vi "DriveSimulationExecute.vi"(6 "GyroStatus":T7, 8 "error in (no error)":errorcluster, 9 "GyroValuesDeg":T8, 10 "ModulePositions":T1[](array[typedef]) {"Angle"."SIN" format="%13.4f"; "Angle"."COS" format="%13.4f"; "Angle"."VALUE" format="%13.4f"}, 11 "ModuleStates":T6[](array[typedef]) {"Angle"."SIN" format="%13.4f"; "Angle"."COS" format="%13.4f"; "Angle"."VALUE" format="%13.4f"}) -> (0 "error out":errorcluster, 1 "outModulePositions":T1[](array[typedef]) {"Angle"."SIN" format="%13.4f"; "Angle"."COS" format="%13.4f"; "Angle"."VALUE" format="%13.4f"}, 2 "SpinMotorDmds":dbl[](array[numeric]), 3 "TravelMotorDmds":dbl[](array[numeric]), 5 "out SWERVE_DRIVE_KINEMATICS":T3 {"SavedModuleStates"."Angle"."SIN" format="%13.4f"; "SavedModuleStates"."Angle"."COS" format="%13.4f"; "SavedModuleStates"."Angle"."VALUE" format="%13.4f"; "PrevCoR"."Y" format="%14.3f"; "PrevCoR"."X" format="%14.3f"; "Modules"."Y" format="%14.3f"; "Modules"."X" format="%14.3f"})   [LabVIEW 2023]
doc: "Execute for Drie\n\nClosed control loop for drive\n\ninput: \n error in (cluster)\n\noutput:\n error out (cluster)"
uses:
  <vilib>/Rock Robotics/WPI/ThirdParty/JAS_Junk/TrajLib/TypeDef/SWERVE_DRIVE_MODULE_STATE.ctl
  <vilib>/Rock Robotics/WPI/ThirdParty/ADI/ADIS16470/Typedef/ADIS16470 Data.ctl
  <vilib>/Rock Robotics/WPI/ThirdParty/ADI/ADIS16470/Typedef/ADIS16470 Status.ctl
  <vilib>/Rock Robotics/WPI/ThirdParty/JAS_Junk/TrajLib/TypeDef/SWERVE_DRIVE_KINEMATICS.ctl
  <vilib>/Analysis/Matrix/Datatypes/RealMatrix.ctl
  <vilib>/Rock Robotics/WPI/ThirdParty/JAS_Junk/TrajLib/TypeDef/TRANSLATION2D.ctl
  <vilib>/Rock Robotics/WPI/ThirdParty/JAS_Junk/TrajLib/LinearFilter_LP_BW1_Execute.vi
  <vilib>/Rock Robotics/WPI/ThirdParty/JAS_Junk/TrajLib/LinearFilter_ResetToValue.vi
  <vilib>/Rock Robotics/WPI/ThirdParty/JAS_Junk/TrajLib/LinearFilter_Calculate.vi
  <vilib>/Rock Robotics/WPI/ThirdParty/JAS_Junk/TrajLib/Conv_Deg_Radians.vi
  <vilib>/Rock Robotics/WPI/ThirdParty/JAS_Junk/TrajLib/Rotation2d_CreateAngle.vi
  <vilib>/Rock Robotics/WPI/ThirdParty/JAS_Junk/TrajLib/VI/Util_GetTime_U32.vi
  <vilib>/Rock Robotics/WPI/ThirdParty/JAS_Junk/TrajLib/Conv_Feet_Meters.vi
  DriveGetMaxSpeed.vi
  <vilib>/Rock Robotics/WPI/ThirdParty/JAS_Junk/TrajLib/SwerveModuleState_Optimize.vi
  <vilib>/Rock Robotics/WPI/ThirdParty/JAS_Junk/TrajLib/ControllerUtil_GetModulusError.vi
  GeneralPurpose/PositionControl.vi
  <vilib>/Rock Robotics/WPI/ThirdParty/JAS_Junk/TrajLib/SimpleMotorFF_New.vi
  <vilib>/Rock Robotics/WPI/ThirdParty/JAS_Junk/TrajLib/SimpleMotorFF_Calculate_CalcAccel.vi
  <vilib>/Rock Robotics/WPI/ThirdParty/JAS_Junk/TrajLib/PIDController_AdvExecute.vi
  <vilib>/Rock Robotics/WPI/ThirdParty/JAS_Junk/TrajLib/PIDController_Pack_AdvLimits.vi
  <vilib>/Rock Robotics/WPI/ThirdParty/JAS_Junk/TrajLib/PIDController_Pack_AdvTuning.vi
  <vilib>/Rock Robotics/WPI/ThirdParty/JAS_Junk/TrajLib/SlewRateLimiter_Execute.vi
  GeneralPurpose/Robot_Enabled.vi
  <vilib>/Rock Robotics/WPI/ThirdParty/JAS_Junk/TrajLib/Rotation2d_Minus.vi
  <vilib>/Rock Robotics/WPI/ThirdParty/JAS_Junk/TrajLib/Rotation2d_GetRadians.vi
  <vilib>/Rock Robotics/WPI/ThirdParty/JAS_Junk/TrajLib/SwerveModuleState_New.vi
  <vilib>/Rock Robotics/WPI/ThirdParty/JAS_Junk/TrajLib/Rotation2d_RotateBy.vi
  <vilib>/Rock Robotics/WPI/ThirdParty/JAS_Junk/TrajLib/SimpleMotorFF_Calculate.vi
  <vilib>/Rock Robotics/WPI/ThirdParty/JAS_Junk/TrajLib/PIDController_AtSetpoint.vi
  <vilib>/Rock Robotics/WPI/ThirdParty/JAS_Junk/TrajLib/PIDController_SetPIDF.vi
  <vilib>/Rock Robotics/WPI/ThirdParty/JAS_Junk/TrajLib/PIDController_SetDerivativeFilter.vi
  <vilib>/Rock Robotics/WPI/ThirdParty/JAS_Junk/TrajLib/PIDController_SetIntegratorRange.vi
  <vilib>/Rock Robotics/WPI/ThirdParty/JAS_Junk/TrajLib/PIDController_SetTolerancePandV.vi
  <vilib>/Rock Robotics/WPI/ThirdParty/JAS_Junk/TrajLib/PIDController_DisableContinousInput.vi
  <vilib>/Rock Robotics/WPI/ThirdParty/JAS_Junk/TrajLib/PIDController_EnableContinousInput.vi
  <vilib>/Rock Robotics/WPI/ThirdParty/JAS_Junk/TrajLib/PIDController_Reset.vi
  <vilib>/Rock Robotics/WPI/ThirdParty/JAS_Junk/TrajLib/PIDController_New.vi
  <vilib>/Rock Robotics/WPI/ThirdParty/JAS_Junk/TrajLib/PIDController_SetOutputLimits.vi
  <vilib>/Rock Robotics/WPI/ThirdParty/JAS_Junk/TrajLib/VI/PIDController_SetIntegratorZone.vi
  <vilib>/Rock Robotics/WPI/ThirdParty/JAS_Junk/TrajLib/SlewRateLimiter_New.vi
  <vilib>/Rock Robotics/WPI/ThirdParty/JAS_Junk/TrajLib/SlewRateLimiter_Reset.vi
  <vilib>/Rock Robotics/WPI/ThirdParty/JAS_Junk/TrajLib/SlewRateLimiter_Calculate.vi
  <vilib>/Rock Robotics/WPI/ThirdParty/JAS_Junk/TrajLib/SlewRateLimiter_SetRate.vi
  <vilib>/Rock Robotics/WPI/ThirdParty/JAS_Junk/TrajLib/Rotation2d_UnaryMinus.vi
  <vilib>/Rock Robotics/WPI/ThirdParty/JAS_Junk/TrajLib/Rotation2d_CreateXY.vi
  <vilib>/Rock Robotics/WPI/ThirdParty/JAS_Junk/TrajLib/PIDController_NewPeriod.vi
  <vilib>/Rock Robotics/WPI/ThirdParty/JAS_Junk/TrajLib/Util_CalcDist.vi
  <vilib>/Rock Robotics/SystemInterfaces/NetworkCommunication/NetComm_UsageReport_report.vi
  DriveGlobal.vi
  <vilib>/Rock Robotics/WPI/ThirdParty/JAS_Junk/TrajLib/LinearFilter_LowPassBW1.vi
  <vilib>/Rock Robotics/WPI/ThirdParty/JAS_Junk/TrajLib/VI/Util_GetTime_U64.vi
  Robot Global Data.vi
  <vilib>/Rock Robotics/WPI/ThirdParty/JAS_Junk/TrajLib/Globals/Util_LibraryGlobals.vi
  <vilib>/Rock Robotics/WPI/ThirdParty/JAS_Junk/TrajLib/PIDController_AdvCalculate_FF_Sp_Pv.vi
  <vilib>/Rock Robotics/WPI/ThirdParty/JAS_Junk/TrajLib/Trajectory_Library.lvlib
  <vilib>/Rock Robotics/WPI/ThirdParty/JAS_Junk/TrajLib/TypeDef/ROTATION2D.ctl
  <vilib>/Rock Robotics/WPI/ThirdParty/JAS_Junk/TrajLib/TypeDef/SWERVE_DRIVE_MODULE_POSITION.ctl
  <vilib>/Analysis/Matrix/NI_Matrix.lvlib
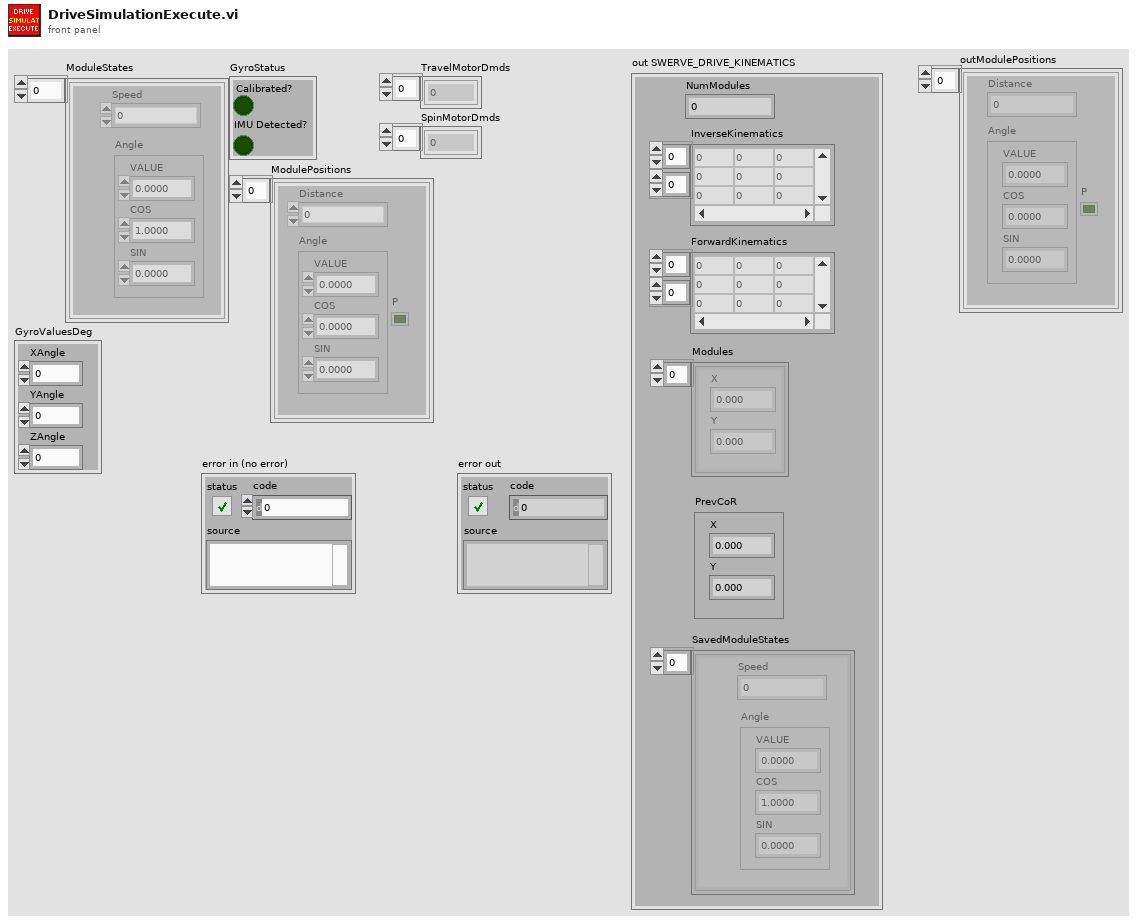
[diagram p1: front panel]
types:
  T1 = typedef "Trajectory_Library.lvlib/SWERVE_DRIVE_MODULE_POSITION.ctl" = cluster{"Distance":dbl, "Angle":T2, "P":bool}
  T2 = typedef "Trajectory_Library.lvlib/ROTATION2D.ctl" = cluster{"VALUE":dbl, "COS":dbl, "SIN":dbl}
  T3 = typedef "Trajectory_Library.lvlib/SWERVE_DRIVE_KINEMATICS.ctl" = cluster{"NumModules":i32, "InverseKinematics":T4, "ForwardKinematics":T4, "Modules":T5[], "PrevCoR":T5, "SavedModuleStates":T6[]}
  T4 = typedef "NI_Matrix.lvlib/RealMatrix.ctl" = dbl[][]
  T5 = typedef "Trajectory_Library.lvlib/TRANSLATION2D.ctl" = cluster{"X":dbl, "Y":dbl}
  T6 = typedef "Trajectory_Library.lvlib/SWERVE_DRIVE_MODULE_STATE.ctl" = cluster{"Speed":dbl, "Angle":T2}
  T7 = typedef "ADIS16470 Status.ctl" = cluster{"Calibrated?":bool, "IMU Detected?":bool}
  T8 = typedef "ADIS16470 Data.ctl" = cluster{"XAngle":dbl, "YAngle":dbl, "ZAngle":dbl}
  T9 = typedef "Trajectory_Library.lvlib/CHASSIS_SPEEDS.ctl" = cluster{"vX":dbl, "vY":dbl, "vOmega":dbl}
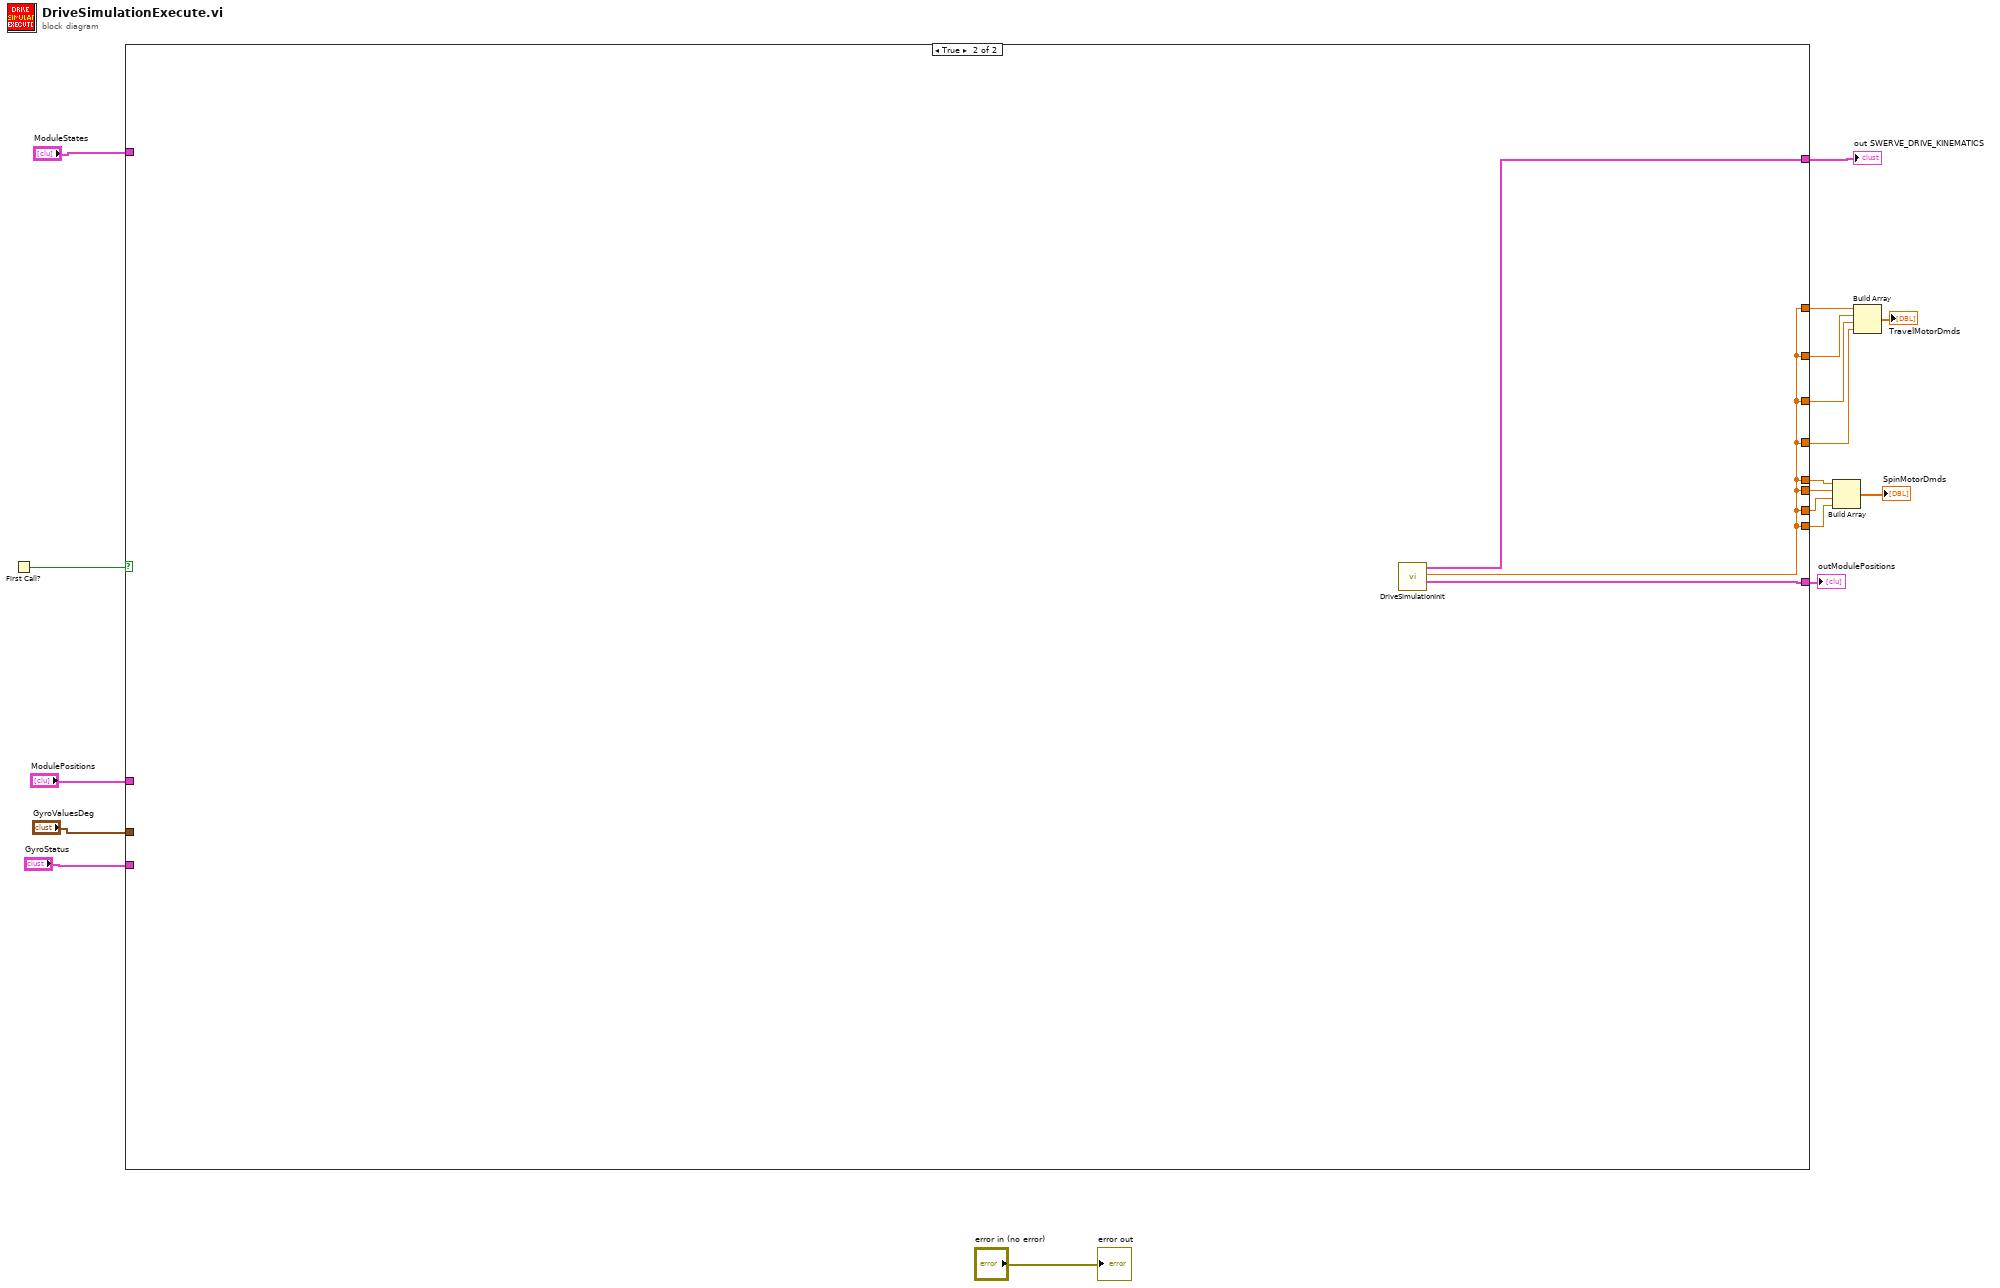
[diagram p0: block diagram]
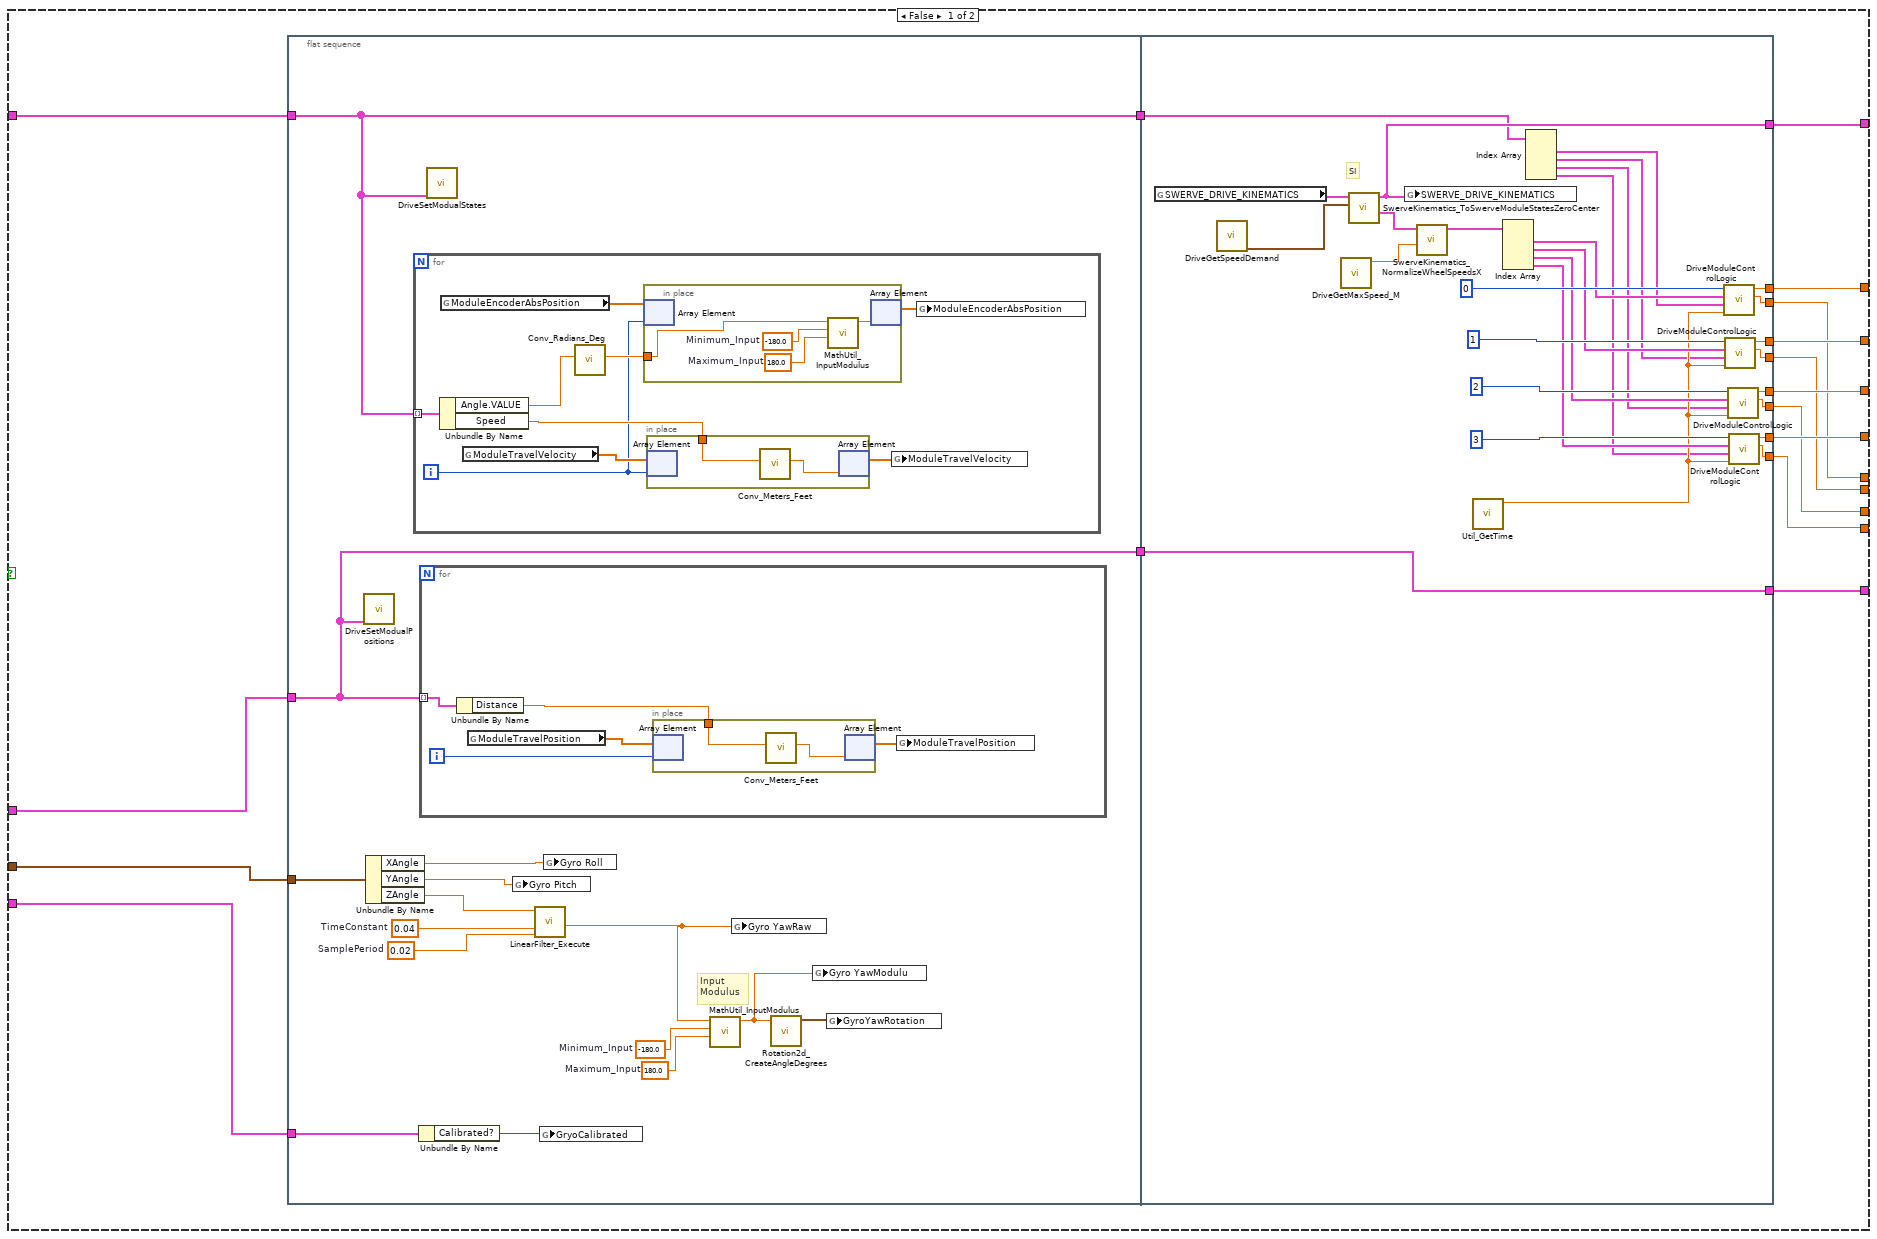
[diagram p2: hidden frame]
diagram:
  n1 = First Call?() -> (First Call?: T/F=w17:bool)
  n2 = case shown="True" w17 {
    tunnel: "ModuleStates" -> [w29 _]
    tunnel: "ModulePositions" -> [w23 _]
    tunnel: "GyroValuesDeg" -> [w22 _]
    tunnel: "GyroStatus" -> [w21 _]
    tunnel: [w28 w103] -> w10
    tunnel: [w26 w103] -> w9
    tunnel: [w25 w103] -> w8
    tunnel: [w24 w103] -> w7
    tunnel: [w34 w103] -> w6
    tunnel: [w33 w103] -> w5
    tunnel: [w32 w103] -> w4
    tunnel: [w31 w103] -> w3
    tunnel: [w30 w102] -> w2
    tunnel: [w20 w101] -> w1
    frame False {
      n3 = flat-sequence {
        tunnel: w29 -> [w49]
        tunnel: [w49] -> w27
        tunnel: w23 -> [w35]
        tunnel: w22 -> [w38]
        tunnel: w21 -> [w36]
        tunnel: [w35] -> w19
        tunnel: [w82] -> w26
        tunnel: [w81] -> w25
        tunnel: [w80] -> w24
        tunnel: [w79] -> w34
        tunnel: [w78] -> w33
        tunnel: [w77] -> w32
        tunnel: [w76] -> w31
        tunnel: [w75] -> w30
        tunnel: [w73] -> w28
        tunnel: w27 -> [w74]
        tunnel: [w72] -> w20
        tunnel: w19 -> [w72]
        frame #0 {
          w41 = -180.0  # Minimum_Input
          w42 = 180.0  # Maximum_Input
          w40 = 0.02  # SamplePeriod
          w39 = 0.04  # TimeConstant
          # "Input\nModulus"
          n4 = call "DriveSetModualPositions.vi"("Swerve_Drive_Modual_Position"=w35) -> ()  [unwired: 11 in]
          n5 = Unbundle By Name(w38) -> ("XAngle"=w48:dbl, "YAngle"=w47:dbl, "ZAngle"=w45:dbl)
          n6 = for {
            tunnel: w49 -> [w63] mode=indexing
            i -> [w58]
            n7 = Unbundle By Name(w63) -> ("Angle.VALUE"=w57:dbl, "Speed"=w62:dbl)
            n8 = global read "DriveGlobal.vi" "ModuleEncoderAbsPosition"() -> (w61:dbl[])
            n9 = global read "DriveGlobal.vi" "ModuleTravelVelocity"() -> (w65:dbl[])
            n10 = call <vilib>:"Conv_Radians_Deg.vi"("Radians"=w57) -> ("Degrees"=w59:dbl)  [unwired: 10 in]
            n11 = in-place {
              in-place-border: w59 -> [w66]
              w69 = -180.0  # Minimum_Input
              w68 = 180.0  # Maximum_Input
              n12 = in-place-array #1(w61, w58) -> ()  [unwired: 1 out]
              n13 = call <vilib>:"MathUtil_InputModulus.vi"("Maximum_Input"=w68, "Minimum_Input"=w69, "Input"=w66) -> ("modulus"=w67:dbl)  [unwired: 8 in]
              n14 = in-place-array #1(w67) -> (w60:dbl[])  [unwired: 1 out]
            }
            n15 = in-place {
              in-place-border: w62 -> [w70]
              n16 = in-place-array #2(w65, w58) -> ()  [unwired: 1 out]
              n17 = call <vilib>:"Conv_Meters_Feet.vi"("Meters"=w70) -> ("Feet"=w71:dbl)  [unwired: 10 in]
              n18 = in-place-array #2(w71) -> (w64:dbl[])  [unwired: 1 out]
            }
            n19 = global write "DriveGlobal.vi" "ModuleTravelVelocity"(w64) -> ()
            n20 = global write "DriveGlobal.vi" "ModuleEncoderAbsPosition"(w60) -> ()
          }
          n21 = Unbundle By Name(w36) -> ("Calibrated?"=w37:bool)
          n22 = for {
            tunnel: w35 -> [w52] mode=indexing
            i -> [w50]
            n23 = Unbundle By Name(w52) -> ("Distance"=w51:dbl)
            n24 = global read "DriveGlobal.vi" "ModuleTravelPosition"() -> (w54:dbl[])
            n25 = in-place {
              in-place-border: w51 -> [w55]
              n26 = in-place-array #3(w54, w50) -> ()  [unwired: 1 out]
              n27 = call <vilib>:"Conv_Meters_Feet.vi"("Meters"=w55) -> ("Feet"=w56:dbl)  [unwired: 10 in]
              n28 = in-place-array #3(w56) -> (w53:dbl[])  [unwired: 1 out]
            }
            n29 = global write "DriveGlobal.vi" "ModuleTravelPosition"(w53) -> ()
          }
          n30 = call "DriveSetModualStates.vi"("Swerve__Drive_Modual_States"=w49) -> ()  [unwired: 11 in]
          n31 = global write "DriveGlobal.vi" "Gyro Pitch"(w47) -> ()
          n32 = call-poly <vilib>:"LinearFilter_Execute.vi"("SamplePeriod"=w40, "TimeConstant"=w39, "Input"=w45) -> ("Output"=w46:dbl)  [unwired: 8 in]
          n33 = global write "DriveGlobal.vi" "GryoCalibrated"(w37) -> ()
          n34 = global write "DriveGlobal.vi" "Gyro Roll"(w48) -> ()
          n35 = call <vilib>:"MathUtil_InputModulus.vi"("Maximum_Input"=w42, "Minimum_Input"=w41, "Input"=w46) -> ("modulus"=w44:dbl)  [unwired: 8 in]
          n36 = global write "DriveGlobal.vi" "Gyro YawRaw"(w46) -> ()
          n37 = call <vilib>:"Rotation2d_CreateAngleDegrees.vi"("Angle_Degrees"=w44) -> ("ROTATION"=w43:T2)  [unwired: 10 in]
          n38 = global write "DriveGlobal.vi" "Gyro YawModulu"(w44) -> ()
          n39 = global write "DriveGlobal.vi" "GyroYawRotation"(w43) -> ()
        }
        frame #1 {
          # "SI"
          n40 = global read "DriveGlobal.vi" "SWERVE_DRIVE_KINEMATICS"() -> (w100:T3)
          n41 = call "DriveGetSpeedDemand.vi"() -> ("ChassisSpeedDemand"=w99:T9)  [unwired: 8 in, 3 out]
          n42 = call "DriveGetMaxSpeed_M.vi"() -> ("Max Speed (m/sec)"=w96:dbl)  [unwired: 11 in]
          n43 = call <vilib>:"SwerveKinematics_ToSwerveModuleStatesZeroCenter.vi"("ChassisSpeeds"=w99, "in SWERVE_DRIVE_KINEMATICS"=w100) -> ("ModuleStates"=w98:T6[], "out SWERVE_DRIVE_KINEMATICS"=w75:T3)  [unwired: 8 in]
          n44 = global write "DriveGlobal.vi" "SWERVE_DRIVE_KINEMATICS"(w75) -> ()
          n45 = call <vilib>:"SwerveKinematics_NormalizeWheelSpeedsX.vi"("AttainableMaxSpeed"=w96, "in WheelStates"=w98) -> ("out WheelStates"=w97:T6[])  [unwired: 9 in]
          n46 = call <vilib>:"Util_GetTime.vi"() -> ("FPGA_Time_Seconds"=w87:dbl)  [unwired: 9 in, 2 out]
          n47 = Index Array(array=w97) -> (element #1=w91:T6, element #2=w90:T6, element #3=w89:T6, element #4=w88:T6)  [unwired: 4 in]
          n48 = Index Array(array=w74) -> (element #1=w86:T6, element #2=w85:T6, element #3=w84:T6, element #4=w83:T6)  [unwired: 4 in]
          n49 = call "DriveModuleControlLogic.vi"("Pass_Through_Time"=w87, "Actual State"=w86, "Desired State"=w91, "ModualNamePrefix"=0) -> ("SpinMotorDmd"=w73:dbl, "TravelMotorDmd"=w79:dbl)  [unwired: 6 in]
          n50 = call "DriveModuleControlLogic.vi"("Pass_Through_Time"=w87, "Actual State"=w85, "Desired State"=w90, "ModualNamePrefix"=1) -> ("SpinMotorDmd"=w82:dbl, "TravelMotorDmd"=w78:dbl)  [unwired: 6 in]
          n51 = call "DriveModuleControlLogic.vi"("Pass_Through_Time"=w87, "Actual State"=w84, "Desired State"=w89, "ModualNamePrefix"=2) -> ("SpinMotorDmd"=w81:dbl, "TravelMotorDmd"=w77:dbl)  [unwired: 6 in]
          n52 = call "DriveModuleControlLogic.vi"("Pass_Through_Time"=w87, "Actual State"=w83, "Desired State"=w88, "ModualNamePrefix"=3) -> ("SpinMotorDmd"=w80:dbl, "TravelMotorDmd"=w76:dbl)  [unwired: 6 in]
        }
      }
    }
    frame True {
      n53 = call "DriveSimulationInit.vi"() -> ("Array"=w101:T1[], "TravelMotorDmd"=w103:dbl, "SWERVE_DRIVE_KINEMATICS"=w102:T3)  [unwired: 9 in]
    }
  }
  "out SWERVE_DRIVE_KINEMATICS" <- w2
  "outModulePositions" <- w1
  n54 = Build Array(w10, w9, w8, w7) -> (→"SpinMotorDmds":dbl[])
  n55 = Build Array(w6, w5, w4, w3) -> (→"TravelMotorDmds":dbl[])
  "error out" <- "error in (no error)"
